vi "Measurement Logic.vi"(8 "error in":errorcluster, 11 "Measurement Configuration":T2={"Load Current in A"=0.005, "Nominal Output Voltage in V"=3.3, "Start"=4.0, "Stop"=6.0, "Step"=0.1, "Input SMU"="", "Load SMU"="", "Input DMM"="", "Load DMM"=""} {"Nominal Output Voltage in V" format="%#_13g"; "Load Current in A" format="%#_13g"}) -> (0 "error out":errorcluster, 3 "Measurement Results":T1)   [LabVIEW 2020, in "Line Regulation.lvlib"]
uses:
  Line Regulation.lvlib
  Reusables/Stimulus And Measure.ctl
  Reusables/Load Output Function.ctl
  Reusables/Prepare Fn Configurations.ctl
  Reusables/Advanced Settings.ctl
  b141144c-5369-402b-8b45-76517362fb79.vi
  TestInputs.ctl
  TestResults.ctl
  Measurement Results.ctl
  Measurement Configuration.ctl
panel:
  out "Line Regulation":cluster{"Iload (mA)":dbl[], "Vout (V)":dbl[]}(graph)
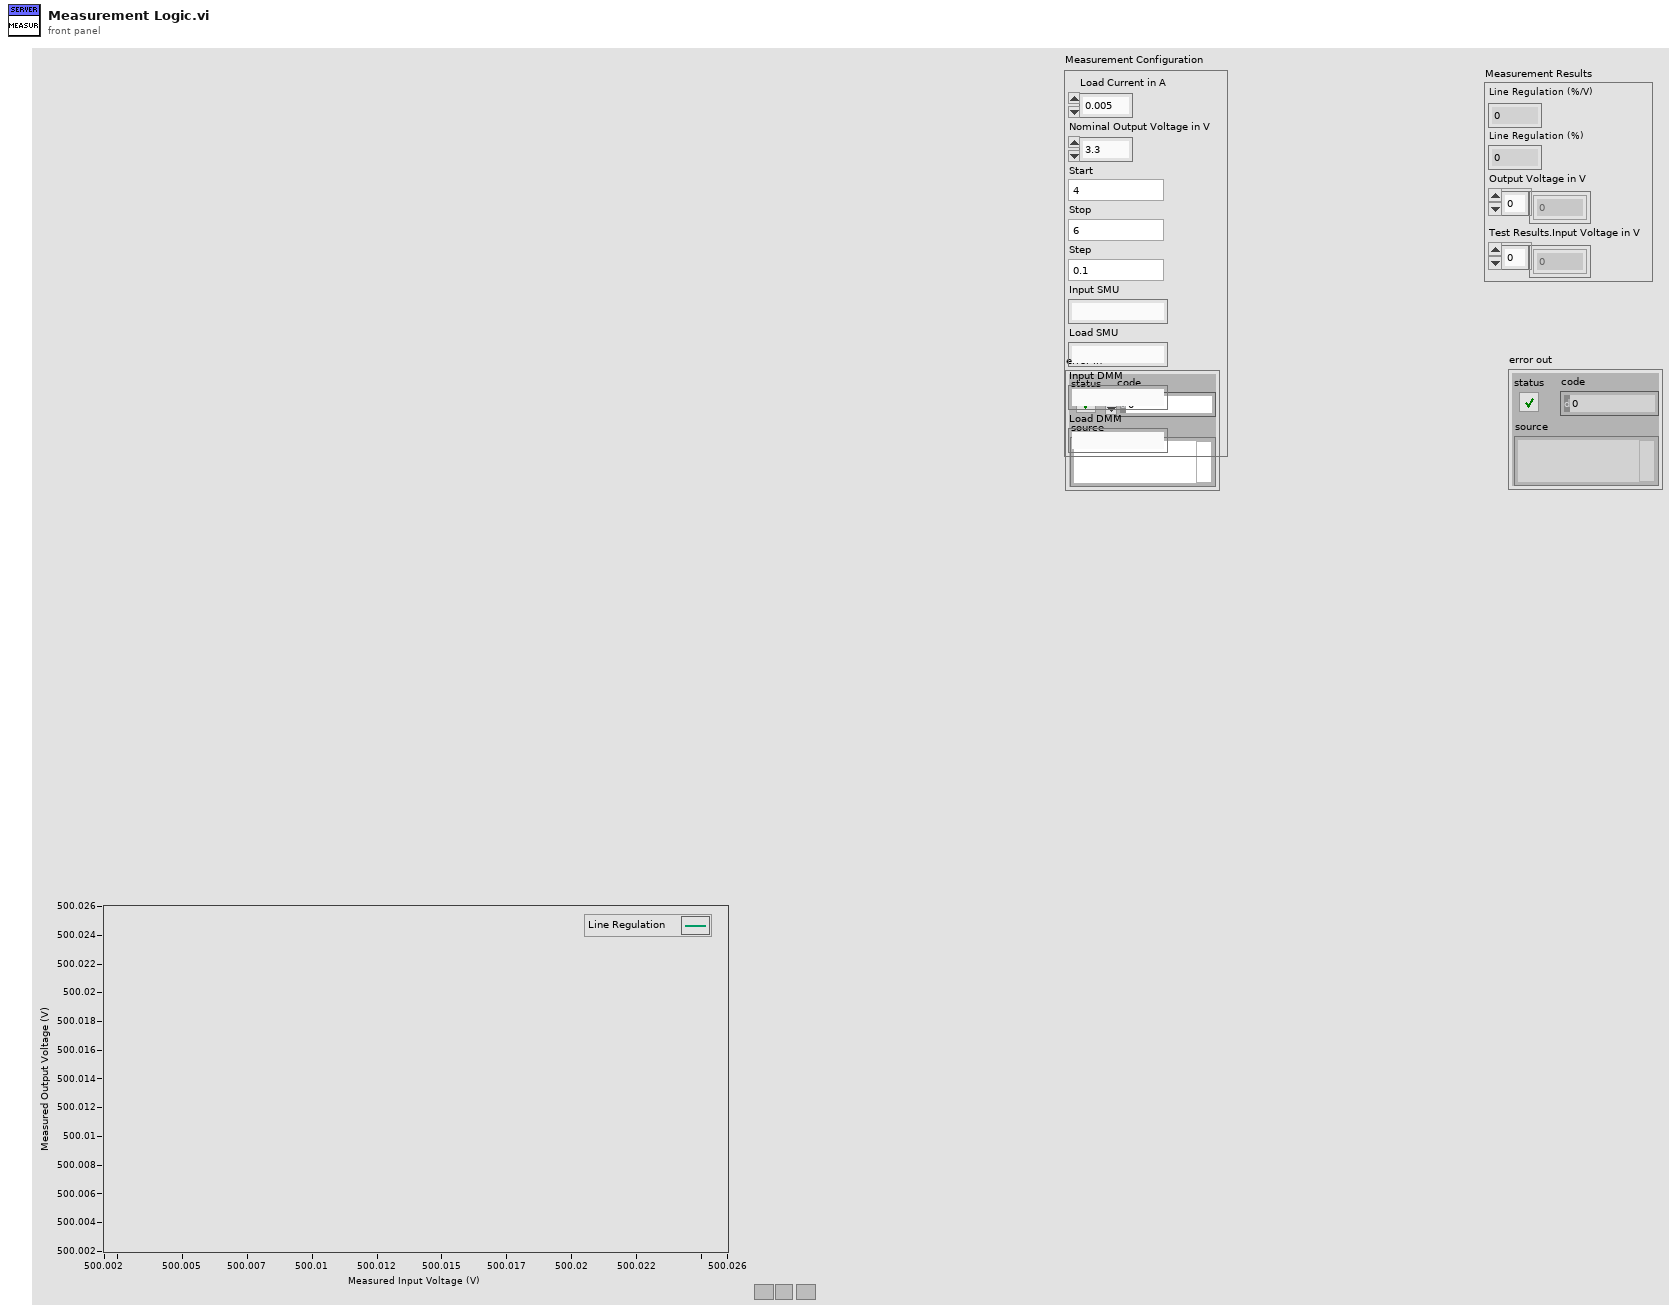
[diagram p1: front panel]
types:
  T1 = typedef "Line Regulation.lvlib/Measurement Results.ctl" = cluster{"Line Regulation (%/V)":dbl, "Line Regulation (%)":dbl, "Output Voltage in V":dbl[], "Test Results.Input Voltage in V":dbl[]}
  T2 = typedef "Line Regulation.lvlib/Measurement Configuration.ctl" = cluster{"Load Current in A":dbl, "Nominal Output Voltage in V":dbl, "Start":dbl, "Stop":dbl, "Step":dbl, "Input SMU":string, "Load SMU":string, "Input DMM":string, "Load DMM":string}
  T3 = typedef "Line Regulation.lvlib/TestInputs.ctl" = cluster{"Load Current in A":dbl, "Input Voltage in V":dbl[], "Nominal Output Voltage in V":dbl, "Advance Setting":T4}
  T4 = typedef "Advanced Settings.ctl" = cluster{"Prepare":T5, "Stimulus And Measure":T7}
  T5 = typedef "Prepare Fn Configurations.ctl" = cluster{"Load SMU Output Function":T6}
  T6 = typedef "Load Output Function.ctl" = enum16{"VoltageSource", "CurrentSource"}
  T7 = typedef "Stimulus And Measure.ctl" = cluster{"Loop Delay in milliSecond":u32}
  T8 = typedef "Line Regulation.lvlib/TestResults.ctl" = cluster{"Input Voltage in V":dbl[], "Input Current in A":dbl[], "Output Voltage in V":dbl[], "Load Current in A":dbl[], "Line Regulation in %/V":dbl, "Line Regulation in %":dbl}
  T9 = cluster{"Test Inputs":T3, "Test Results":T8, "Test Results[][]":string[][], "SMU V":refnum<k15>, "Input DMM":refnum<k15>, "Load DMM":refnum<k15>, "SMU I":refnum<k15>}
  T10 = cluster{"Input Voltage in V":dbl[], "Output Voltage in V":dbl[]}
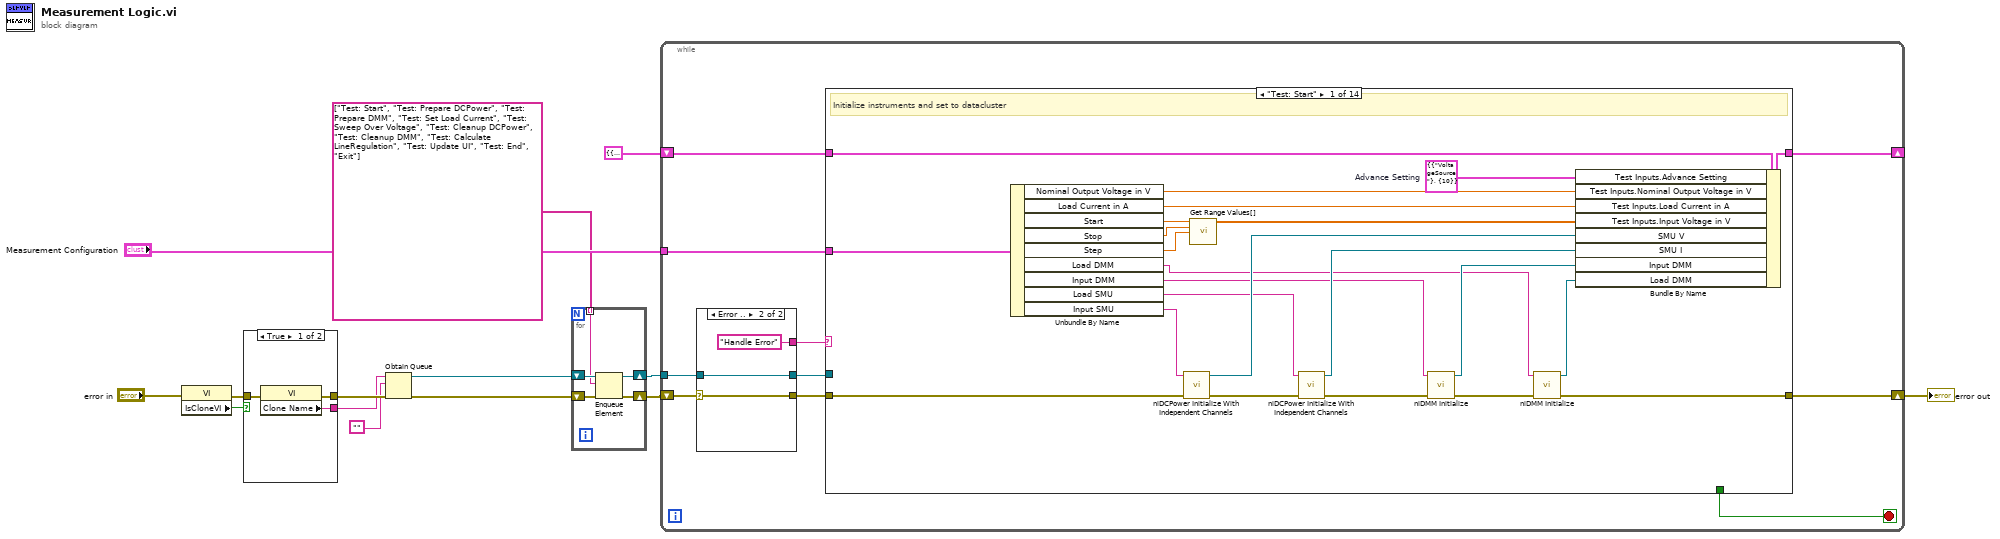
[diagram p0: block diagram]
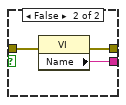
[diagram p2: hidden frame]
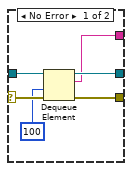
[diagram p3: hidden frame]
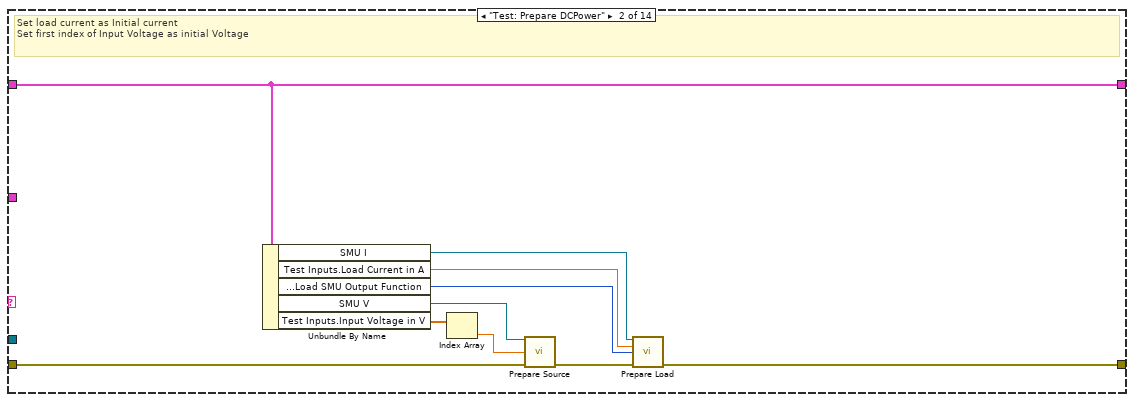
[diagram p4: hidden frame]
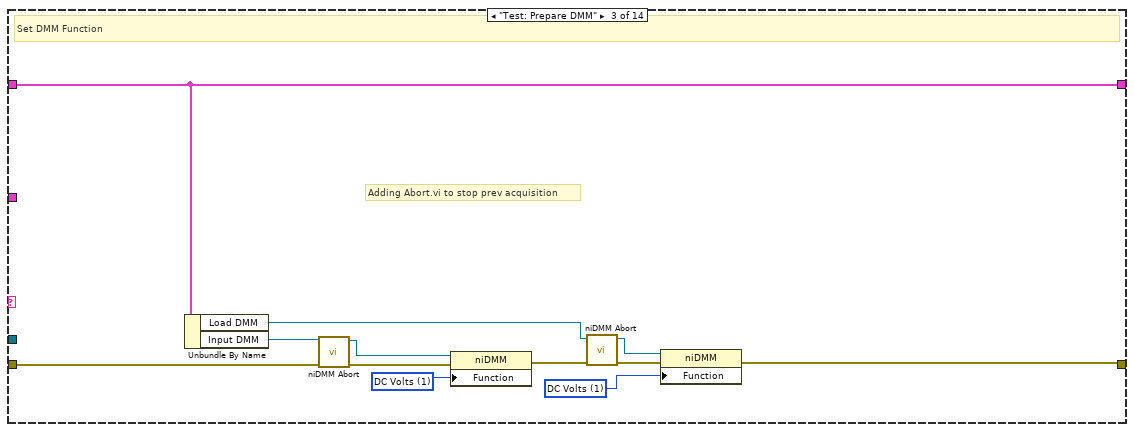
[diagram p5: hidden frame]
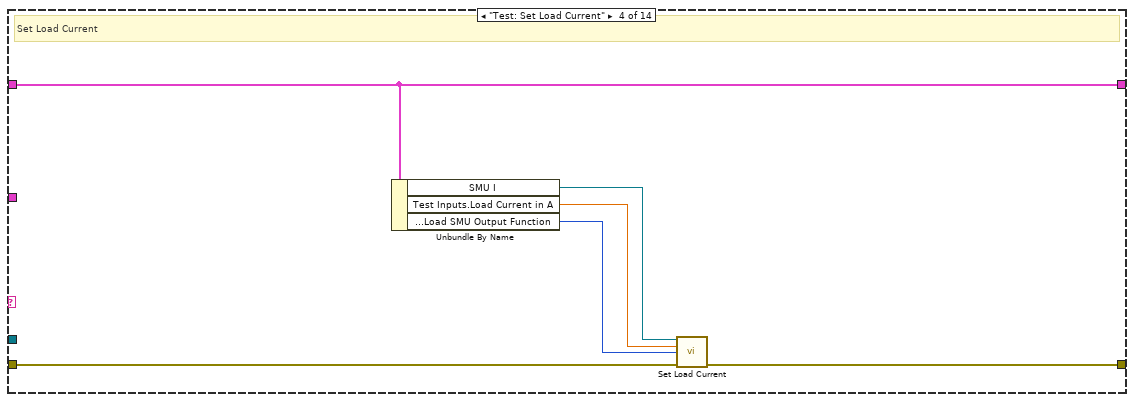
[diagram p6: hidden frame]
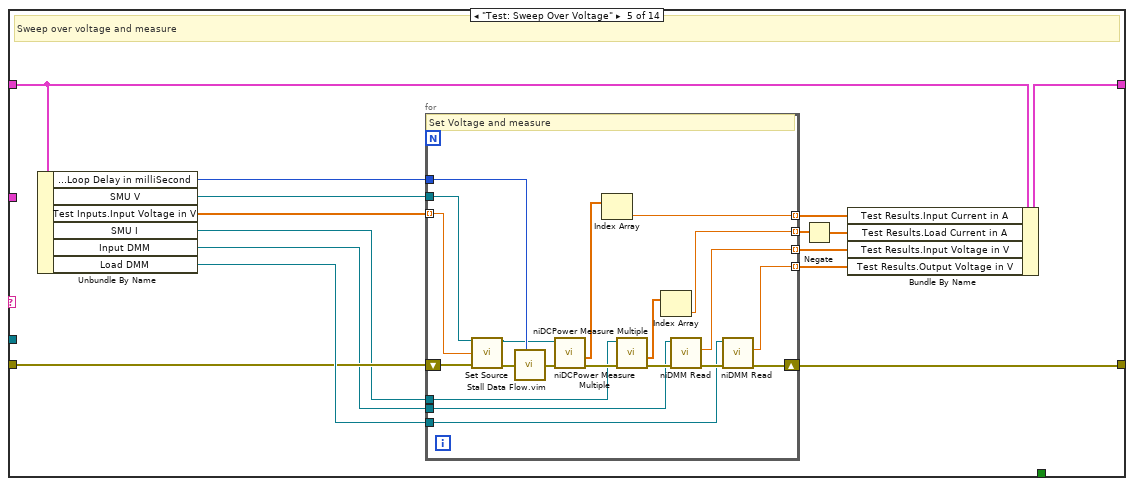
[diagram p7: hidden frame]
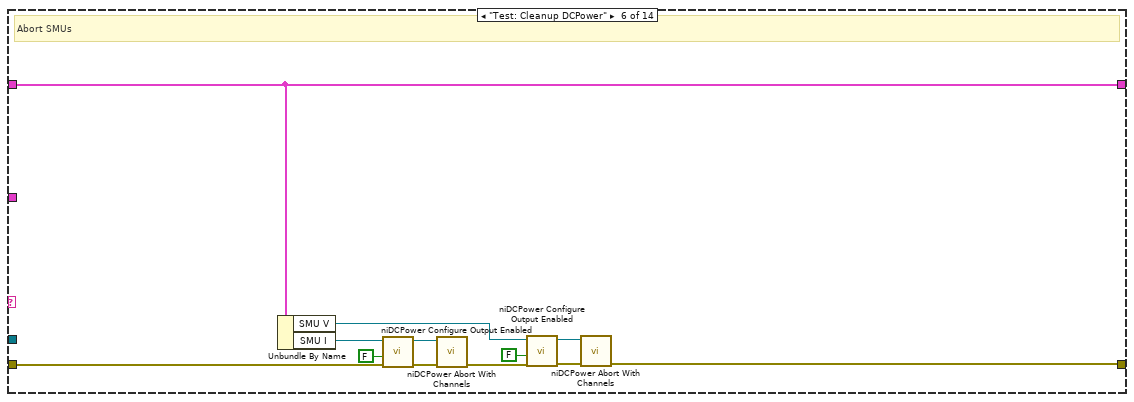
[diagram p8: hidden frame]
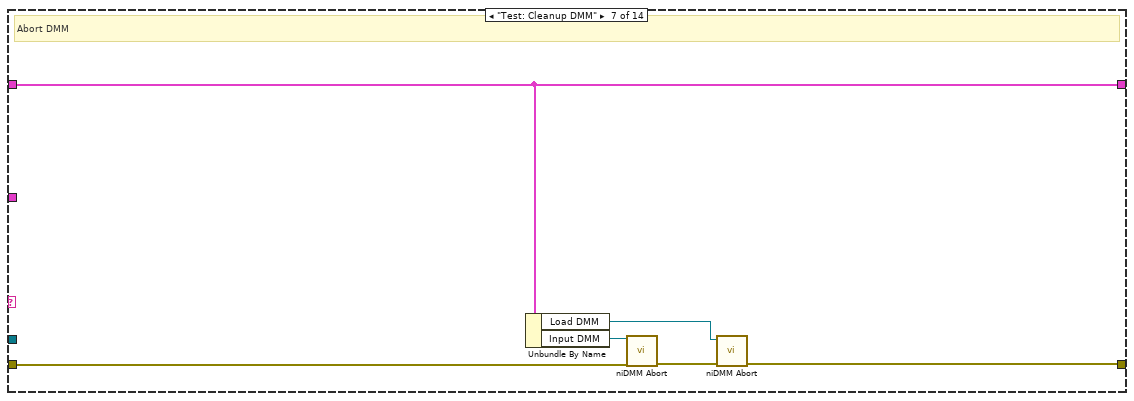
[diagram p9: hidden frame]
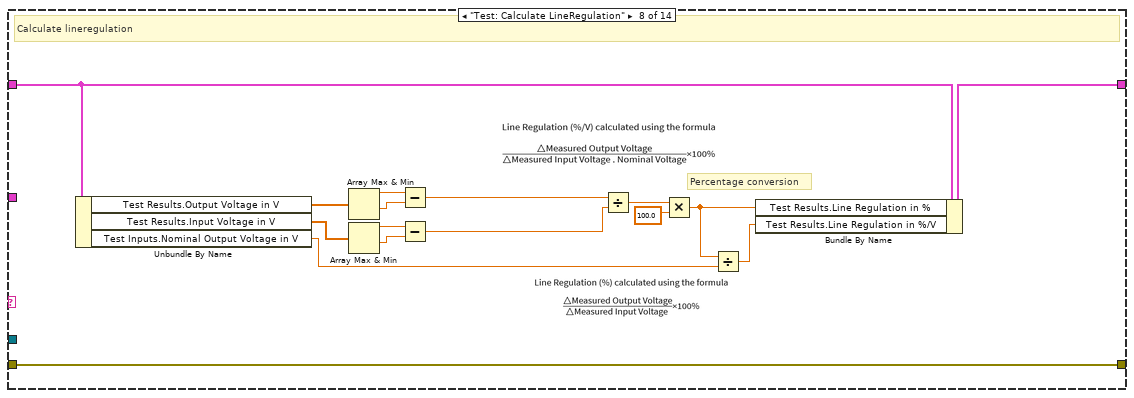
[diagram p10: hidden frame]
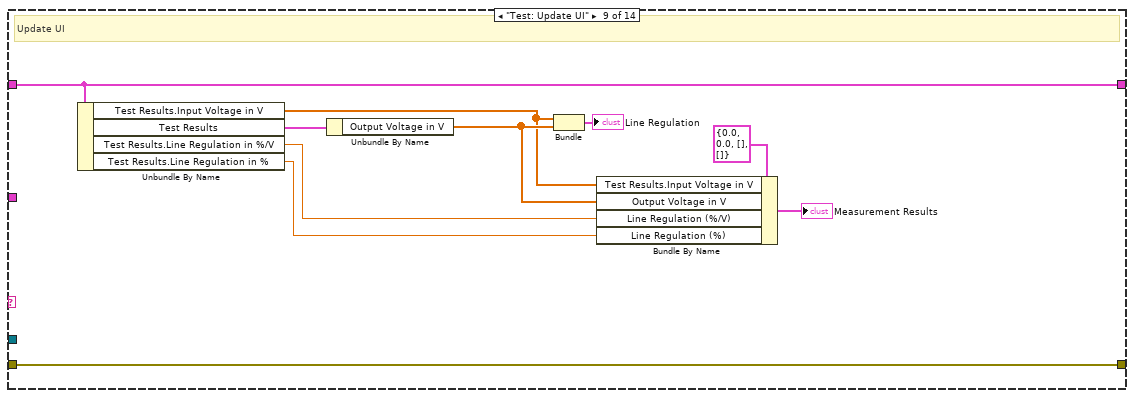
[diagram p11: hidden frame]
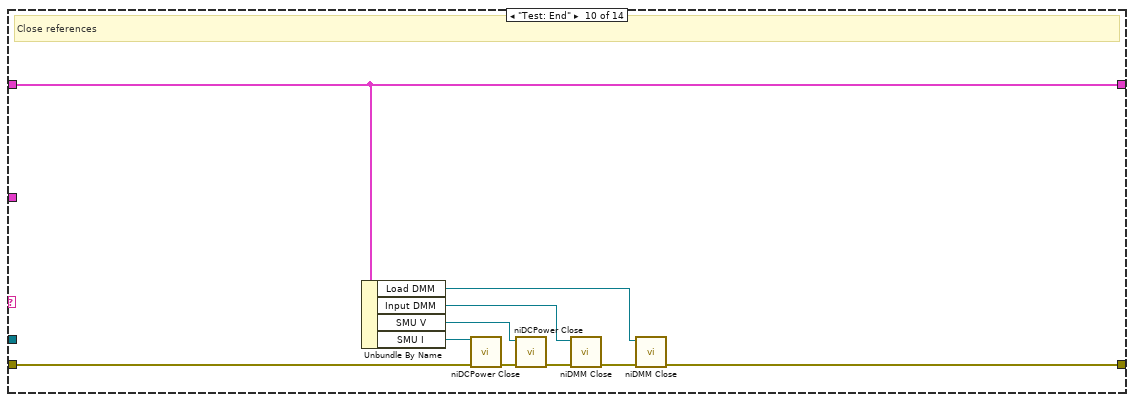
[diagram p12: hidden frame]
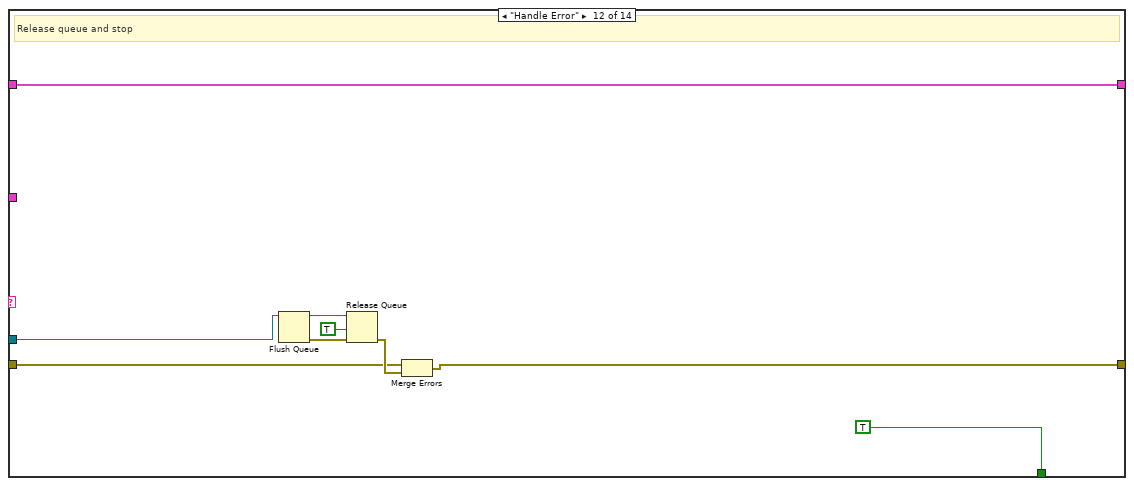
[diagram p14: hidden frame]
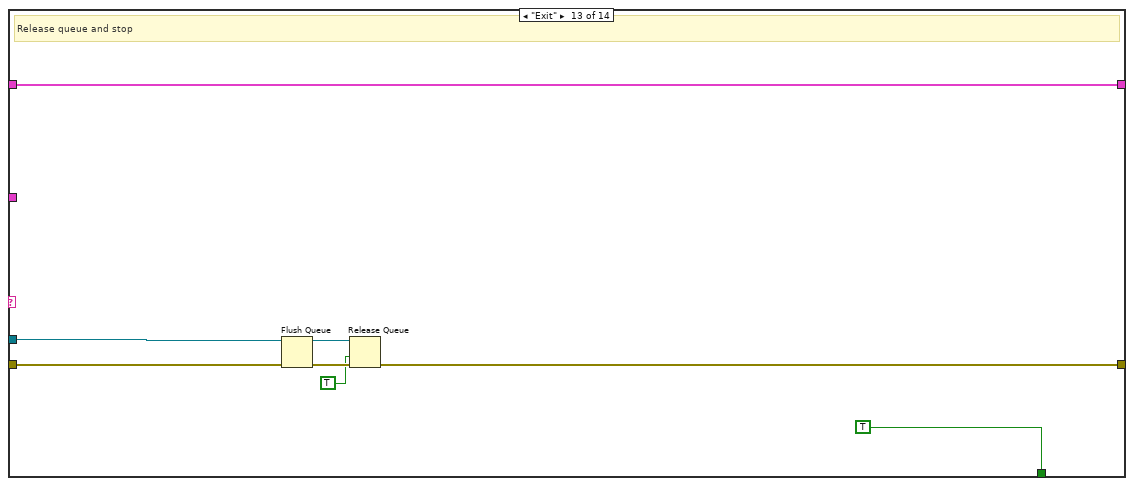
[diagram p15: hidden frame]
diagram:
  n1 = property class="VI"(error in="error in") -> (error out=w7:errorcluster, "IsCloneVI"=w8:bool)  [unwired: 1 in, 1 out]
  n2 = case shown="True" w8 {
    tunnel: [w17 w20] -> w13
    tunnel: [w16 w19] -> w12
    tunnel: w7 -> [w15 w18]
    frame True {
      n3 = property class="VI"(error in=w15) -> (error out=w17:errorcluster, "Clone Name"=w16:string)  [unwired: 1 in, 1 out]
    }
    frame False {
      n4 = property class="VI"(error in=w18) -> (error out=w20:errorcluster, "Name"=w19:string)  [unwired: 1 in, 1 out]
    }
  }
  n5 = Obtain Queue(name (unnamed)=w12, element data type="", error in (no error)=w13) -> (queue out=w10:refnum<queue>, error out=w11:errorcluster)  [unwired: 2 in, 1 out]
  n6 = for {
    shift-right: [w23] -> w6
    shift-left: w11 -> [w25]
    shift-right: [w22] -> w5
    shift-left: w10 -> [w24]
    tunnel: string[] ["Test: Start", "Test: Prepare DCPower", "Test: Prepare DMM", "Test: Set Load Current", "Test: Sweep Over Voltage", "Test: Cleanup DCPower", "Test: Cleanup DMM", "Test: Calculate LineRegulation", "Test: Update UI", "Test: End", "Exit"] -> [w21] mode=indexing
    n7 = Enqueue Element(queue=w24, element=w21, error in (no error)=w25) -> (queue out=w22:refnum<queue>, error out=w23:errorcluster)  [unwired: 1 in, 1 out]
  }
  n8 = while {
    shift-right: [w35] -> w1
    shift-left: w6 -> [w31]
    shift-right: [w33] -> _
    shift-left: T9 {"Test Inputs"={"Load Current in A"=0.0, "Input Voltage in V"=[], "Nominal Output Voltage in V"=0.0, "Advance Setting"={"Prepare"={"Load SMU Output Function"=enum."VoltageSource"}, "Stimulus And Measure"={"Loop Delay in milliSecond"=1}}}, "Test Results"={"Input Voltage in V"=[], "Input Current in A"=[], "Output Voltage in V"=[], "Load Current in A"=[], "Line Regulation in %/V"=0.0, "Line Regulation in %"=0.0}, "Test Results[][]"=[], "SMU V"="", "Input DMM"="", "Load DMM"="", "SMU I"=""} -> [w34]
    tunnel: w5 -> [w27]
    tunnel: "Measurement Configuration" -> [w26]
    stop <- w32 stop-if-true
    n9 = case shown="Error .." w31 {
      selector: w31 -> [w41 w44]
      tunnel: [w40 w44] -> w28
      tunnel: w27 -> [w39 w43]
      tunnel: [w38 w43] -> w30
      tunnel: [w37 "Handle Error"] -> w29
      frame No Error {
        n10 = Dequeue Element(queue=w39, timeout in ms (-1)=100, error in (no error)=w41) -> (queue out=w38:refnum<queue>, element=w37:string, error out=w40:errorcluster)  [unwired: 1 out]
      }
      frame Error {
      }
    }
    n11 = case shown="\"Test: Start\"" w29 {
      tunnel: w30 -> [_ _ _ _ _ _ _ _ _ _ _ w189 w196 _]
      tunnel: w28 -> [w50 w70 w78 w92 w98 w131 w143 w149 w167 w175 w186 w187 w198 w204]
      tunnel: [w49 w71 w80 w93 w101 w139 w146 w149 w167 w178 w186 w194 w197 w204] -> w35
      tunnel: w34 -> [w66 w76 w86 w95 w99 w138 w148 w150 w172 w184 w185 w195 w203 w205]
      tunnel: [w67 w76 w86 w95 w100 w138 w148 w151 w172 w184 w185 w195 w203 w205] -> w33
      tunnel: [_ _ _ _ _ _ _ _ _ _ _ TRUE TRUE _] -> w32
      tunnel: w26 -> [w45 _ _ _ _ _ _ _ _ _ _ _ _ _]
      frame "Test: Start" {
        w46 = T4 {"Prepare"={"Load SMU Output Function"=enum."VoltageSource"}, "Stimulus And Measure"={"Loop Delay in milliSecond"=10}}  # Advance Setting
        # "Initialize instruments and set to datacluster"
        n12 = Unbundle By Name(w45) -> ("Nominal Output Voltage in V"=w48:dbl, "Load Current in A"=w47:dbl, "Start"=w58:dbl, "Stop"=w57:dbl, "Step"=w56:dbl, "Load DMM"=w54:string, "Input DMM"=w53:string, "Load SMU"=w52:string, "Input SMU"=w51:string)
        n13 = call <instrlib>:"niDCPower Initialize With Independent Channels.vi"("error in (no error)"=w50, "resource name"=w51) -> ("error out"=w62:errorcluster, "instrument handle out"=w65:refnum<k15>)  [unwired: 8 in]
        n14 = call "Get Range Values[].vi"("Start"=w58, "Stop"=w57, "Step Size"=w56) -> ("Values[]"=w55:dbl[])  [unwired: 12 in]
        n15 = call <instrlib>:"niDCPower Initialize With Independent Channels.vi"("error in (no error)"=w62, "resource name"=w52) -> ("error out"=w61:errorcluster, "instrument handle out"=w59:refnum<k15>)  [unwired: 8 in]
        n16 = call <instrlib>:"niDMM Initialize.vi"("error in (no error)"=w61, "Instrument Descriptor"=w53) -> ("error out"=w63:errorcluster, "instrument handle out"=w60:refnum<k15>)  [unwired: 8 in]
        n17 = call <instrlib>:"niDMM Initialize.vi"("error in (no error)"=w63, "Instrument Descriptor"=w54) -> ("error out"=w49:errorcluster, "instrument handle out"=w64:refnum<k15>)  [unwired: 8 in]
        n18 = Bundle By Name(cluster=w66, "Test Inputs.Advance Setting"=w46, "Test Inputs.Nominal Output Voltage in V"=w48, "Test Inputs.Load Current in A"=w47, "Test Inputs.Input Voltage in V"=w55, "SMU V"=w65, "SMU I"=w59, "Input DMM"=w60, "Load DMM"=w64) -> (w67:T9)
      }
      frame "Test: Prepare DCPower" {
        # "Set load current as Initial current\nSet first index of Input Voltage as initial Voltage"
        n19 = Unbundle By Name(w76) -> ("SMU I"=w73:refnum<k15>, "Test Inputs.Load Current in A"=w69:dbl, "Test Inputs.Advance Setting.Prepare.Load SMU Output Function"=w68:T6, "SMU V"=w75:refnum<k15>, "Test Inputs.Input Voltage in V"=w77:dbl[])
        n20 = Index Array(array=w77) -> (element=w74:dbl)  [unwired: 1 in]
        n21 = call "Prepare Source.vi"("instrument handle"=w75, "Initial Voltage Level (V)"=w74, "error in (no error)"=w70) -> ("error out"=w72:errorcluster)  [unwired: 12 in]
        n22 = call "Prepare Load.vi"("instrument handle"=w73, "Load Current Level (A)"=w69, "Load Output Function"=w68, "error in (no error)"=w72) -> ("error out"=w71:errorcluster)  [unwired: 11 in]
      }
      frame "Test: Prepare DMM" {
        w82 = 1 items=["DC Volts"=1, "AC Volts"=2, "DC Current"=3, "AC Current"=4, "2-Wire Resistance"=5, "4-Wire Resistance"=101, "Frequency"=104, "Period"=105, "AC Volts DC Coupled"=1001, "Diode"=1002, "Waveform Voltage"=1003, "Waveform Current"=1004, "Capacitance"=1005, "Inductance"=1006, "Temperature"=108] ("Configuration:Function")
        w89 = 1 items=["DC Volts"=1, "AC Volts"=2, "DC Current"=3, "AC Current"=4, "2-Wire Resistance"=5, "4-Wire Resistance"=101, "Frequency"=104, "Period"=105, "AC Volts DC Coupled"=1001, "Diode"=1002, "Waveform Voltage"=1003, "Waveform Current"=1004, "Capacitance"=1005, "Inductance"=1006, "Temperature"=108] ("Configuration:Function")
        # "Adding Abort.vi to stop prev acquisition"
        # "Set DMM Function"
        n23 = Unbundle By Name(w86) -> ("Load DMM"=w79:refnum<k15>, "Input DMM"=w85:refnum<k15>)
        n24 = call <instrlib>:"niDMM Abort.vi"("error in (no error)"=w78, "instrument handle"=w85) -> ("error out"=w88:errorcluster, "instrument handle out"=w87:refnum<k15>)  [unwired: 8 in]
        n25 = property class="niDMM"(reference=w87, error in=w88, "Function"=w89) -> (error out=w81:errorcluster)  [unwired: 1 out]
        n26 = call <instrlib>:"niDMM Abort.vi"("error in (no error)"=w81, "instrument handle"=w79) -> ("error out"=w83:errorcluster, "instrument handle out"=w84:refnum<k15>)  [unwired: 8 in]
        n27 = property class="niDMM"(reference=w84, error in=w83, "Function"=w82) -> (error out=w80:errorcluster)  [unwired: 1 out]
      }
      frame "Test: Set Load Current" {
        # "Set Load Current"
        n28 = Unbundle By Name(w95) -> ("SMU I"=w94:refnum<k15>, "Test Inputs.Load Current in A"=w91:dbl, "Test Inputs.Advance Setting.Prepare.Load SMU Output Function"=w90:T6)
        n29 = call "Set Load Current.vi"("instrument handle in"=w94, "current level"=w91, "OutputFunction"=w90, "error in (no error)"=w92) -> ("error out"=w93:errorcluster)  [unwired: 10 in, 1 out]
      }
      frame "Test: Sweep Over Voltage" {
        # "Sweep over voltage and measure"
        n30 = Unbundle By Name(w99) -> ("Test Inputs.Advance Setting.Stimulus And Measure.Loop Delay in milliSecond"=w108:u32, "SMU V"=w110:refnum<k15>, "Test Inputs.Input Voltage in V"=w109:dbl[], "SMU I"=w96:refnum<k15>, "Input DMM"=w97:refnum<k15>, "Load DMM"=w107:refnum<k15>)
        n31 = for {
          tunnel: w110 -> [w129]
          tunnel: w109 -> [w128] mode=indexing
          tunnel: w108 -> [w126]
          tunnel: w97 -> [w119]
          tunnel: w107 -> [w118]
          tunnel: [w117] -> w105 mode=indexing
          tunnel: [w116] -> w104 mode=indexing
          tunnel: [w115] -> w103 mode=indexing
          tunnel: [w114] -> w102 mode=indexing
          shift-right: [w113] -> w101
          shift-left: w98 -> [w130]
          tunnel: w96 -> [w111]
          # "Set Voltage and measure"
          n32 = call "Set Source.vi"("instrument handle in"=w129, "Vin in V"=w128, "error in (no error)"=w130) -> ("instrument handle out"=w112:refnum<k15>, "error out"=w127:errorcluster)  [unwired: 11 in]
          n33 = call "Stall Data Flow.vim"("value in"=w127, "milliseconds to wait"=w126) -> ("value out"=w120:errorcluster)  [unwired: 1 out]
          n34 = call <instrlib>:"niDCPower Measure Multiple.vi"("error in (no error)"=w120, "instrument handle"=w112) -> ("error out"=w122:errorcluster, "current measurements"=w125:dbl[])  [unwired: 6 in, 2 out]
          n35 = Index Array(array=w125) -> (element=w117:dbl)  [unwired: 1 in]
          n36 = call <instrlib>:"niDCPower Measure Multiple.vi"("error in (no error)"=w122, "instrument handle"=w111) -> ("error out"=w121:errorcluster, "current measurements"=w123:dbl[])  [unwired: 6 in, 2 out]
          n37 = Index Array(array=w123) -> (element=w116:dbl)  [unwired: 1 in]
          n38 = call <instrlib>:"niDMM Read.vi"("error in (no error)"=w121, "instrument handle"=w119) -> ("error out"=w124:errorcluster, "Measurement"=w115:dbl)  [unwired: 7 in, 1 out]
          n39 = call <instrlib>:"niDMM Read.vi"("error in (no error)"=w124, "instrument handle"=w118) -> ("error out"=w113:errorcluster, "Measurement"=w114:dbl)  [unwired: 7 in, 1 out]
        }
        n40 = Negate(x=w104) -> (-x=w106:dbl[])
        n41 = Bundle By Name(cluster=w99, "Test Results.Input Current in A"=w105, "Test Results.Load Current in A"=w106, "Test Results.Input Voltage in V"=w103, "Test Results.Output Voltage in V"=w102) -> (w100:T9)
      }
      frame "Test: Cleanup DCPower" {
        # "Abort SMUs"
        n42 = Unbundle By Name(w138) -> ("SMU V"=w137:refnum<k15>, "SMU I"=w132:refnum<k15>)
        n43 = call <instrlib>:"niDCPower Configure Output Enabled.vi"("error in (no error)"=w131, "output enabled"=FALSE, "instrument handle"=w132) -> ("error out"=w133:errorcluster, "instrument handle out"=w136:refnum<k15>)  [unwired: 7 in]
        n44 = call <instrlib>:"niDCPower Abort With Channels.vi"("error in (no error)"=w133, "instrument handle"=w136) -> ("error out"=w134:errorcluster)  [unwired: 8 in, 1 out]
        n45 = call <instrlib>:"niDCPower Configure Output Enabled.vi"("error in (no error)"=w134, "output enabled"=FALSE, "instrument handle"=w137) -> ("error out"=w141:errorcluster, "instrument handle out"=w140:refnum<k15>)  [unwired: 7 in]
        n46 = call <instrlib>:"niDCPower Abort With Channels.vi"("error in (no error)"=w141, "instrument handle"=w140) -> ("error out"=w139:errorcluster)  [unwired: 8 in, 1 out]
      }
      frame "Test: Cleanup DMM" {
        # "Abort DMM"
        n47 = Unbundle By Name(w148) -> ("Load DMM"=w145:refnum<k15>, "Input DMM"=w144:refnum<k15>)
        n48 = call <instrlib>:"niDMM Abort.vi"("error in (no error)"=w143, "instrument handle"=w144) -> ("error out"=w147:errorcluster)  [unwired: 8 in, 1 out]
        n49 = call <instrlib>:"niDMM Abort.vi"("error in (no error)"=w147, "instrument handle"=w145) -> ("error out"=w146:errorcluster)  [unwired: 8 in, 1 out]
      }
      frame "Test: Calculate LineRegulation" {
        # "Percentage conversion"
        # "Calculate lineregulation"
        n50 = Unbundle By Name(w150) -> ("Test Results.Output Voltage in V"=w162:dbl[], "Test Results.Input Voltage in V"=w157:dbl[], "Test Inputs.Nominal Output Voltage in V"=w153:dbl)
        n51 = Array Max & Min(array=w162) -> (max value=w164:dbl, min value=w160:dbl)  [unwired: 2 out]
        n52 = Array Max & Min(array=w157) -> (max value=w158:dbl, min value=w159:dbl)  [unwired: 2 out]
        n53 = Subtract(x=w164, y=w160) -> (x-y=w161:dbl)
        n54 = Subtract(x=w158, y=w159) -> (x-y=w156:dbl)
        n55 = Divide(x=w161, y=w156) -> (x/y=w155:dbl)
        n56 = Multiply(x=w155, y=100.0) -> (x*y=w154:dbl)
        n57 = Divide(x=w154, y=w153) -> (x/y=w152:dbl)
        n58 = Bundle By Name(cluster=w150, "Test Results.Line Regulation in %"=w154, "Test Results.Line Regulation in %/V"=w152) -> (w151:T9)
      }
      frame "Test: Update UI" {
        # "Update UI"
        n59 = Unbundle By Name(w172) -> ("Test Results.Input Voltage in V"=w168:dbl[], "Test Results"=w173:T8, "Test Results.Line Regulation in %/V"=w171:dbl, "Test Results.Line Regulation in %"=w170:dbl)
        n60 = Unbundle By Name(w173) -> ("Output Voltage in V"=w169:dbl[])
        n61 = Bundle("Input Voltage in V"=w168, "Output Voltage in V"=w169) -> (→"Line Regulation":T10)  [unwired: 1 in]
        n62 = Bundle By Name(cluster=T1 {"Line Regulation (%/V)"=0.0, "Line Regulation (%)"=0.0, "Output Voltage in V"=[], "Test Results.Input Voltage in V"=[]} ("Measurement Results"), "Test Results.Input Voltage in V"=w168, "Output Voltage in V"=w169, "Line Regulation (%/V)"=w171, "Line Regulation (%)"=w170) -> (→"Measurement Results":T1)
      }
      frame "Test: End" {
        # "Close references"
        n63 = Unbundle By Name(w184) -> ("Load DMM"=w179:refnum<k15>, "Input DMM"=w180:refnum<k15>, "SMU V"=w183:refnum<k15>, "SMU I"=w177:refnum<k15>)
        n64 = call <instrlib>:"niDCPower Close.vi"("error in (no error)"=w175, "instrument handle"=w177) -> ("error out"=w176:errorcluster)  [unwired: 9 in]
        n65 = call <instrlib>:"niDCPower Close.vi"("error in (no error)"=w176, "instrument handle"=w183) -> ("error out"=w182:errorcluster)  [unwired: 9 in]
        n66 = call <instrlib>:"niDMM Close.vi"("error in (no error)"=w182, "instrument handle"=w180) -> ("error out"=w181:errorcluster)  [unwired: 9 in]
        n67 = call <instrlib>:"niDMM Close.vi"("error in (no error)"=w181, "instrument handle"=w179) -> ("error out"=w178:errorcluster)  [unwired: 9 in]
      }
      frame "----Misc------" {
      }
      frame "Handle Error" {
        # "Release queue and stop"
        n68 = Flush Queue(queue=w189) -> (queue out=w192:refnum<queue>, error out=w191:errorcluster)  [unwired: 1 in, 1 out]
        n69 = Release Queue(queue=w192, force destroy? (F)=TRUE, error in (no error)=w191) -> (error out=w188:errorcluster)  [unwired: 2 out]
        n70 = Merge Errors(w187, w188) -> (w194:errorcluster)
      }
      frame "Exit" {
        # "Release queue and stop"
        n71 = Flush Queue(queue=w196, error in (no error)=w198) -> (queue out=w201:refnum<queue>, error out=w200:errorcluster)  [unwired: 1 out]
        n72 = Release Queue(queue=w201, force destroy? (F)=TRUE, error in (no error)=w200) -> (error out=w197:errorcluster)  [unwired: 2 out]
      }
      frame "", Default {
        # "Do nothing"
      }
    }
  }
  "error out" <- w1
